vi "Create ObjectList.vi"(5 "ObjectList in":refnum<class "ObjectList.lvclass">, 7 "List Implementation (Array)":refnum<class "ListImp.lvclass">, 8 "error in (no error)":errorcluster) -> (0 "error out":errorcluster, 3 "ObjectList":refnum<class "ObjectList.lvclass">)   [LabVIEW 2013, in "LapDog.Collections.v_.Lists.lvlib" / "ObjectList.lvclass"]
doc: "Creates a List object. Wire a List Implementation object cube to the List Implementation input terminal to use an implementation other than the default array implementation. This method will automatically invoke the Create method for the implementation object.\n\nThis method returns a default List object if an error is on the input terminal."
uses:
  ObjectList.lvclass
  ListImp/ListImp.lvclass
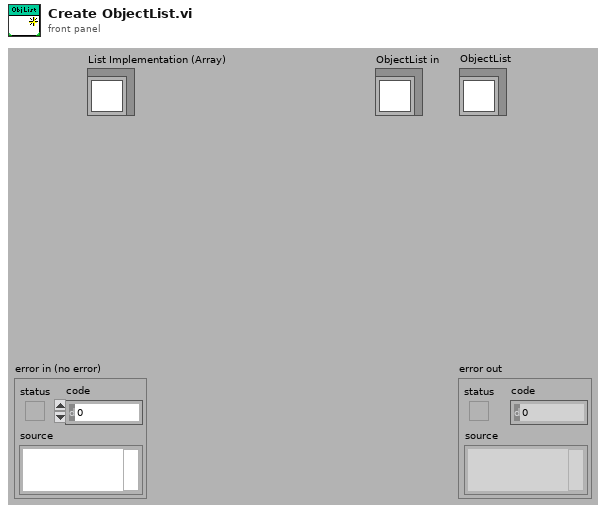
[diagram p1: front panel]
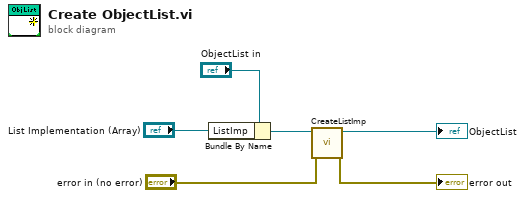
[diagram p0: block diagram]
diagram:
  n1 = Bundle By Name(cluster="ObjectList in", "ListImp"="List Implementation (Array)") -> (w4:refnum<class "ObjectList.lvclass">)
  n2 = call "CreateListImp.vi"("error in (no error)"="error in (no error)", "List in"=w4) -> ("error out"=→"error out":errorcluster, "List out"=→"ObjectList":refnum<class "ObjectList.lvclass">)  [unwired: 8 in]
